vi "Check for Value Changes.vi"(8 "error in (no error)":errorcluster, 11 "Settings in":refnum<class "Settings.lvclass">) -> (0 "error out":errorcluster, 2 "Changes have been made":bool, 3 "Settings out":refnum<class "Settings.lvclass">)   [LabVIEW 2017, in "Settings.lvclass"]
uses:
  Settings.lvclass
  Settings.lvclass/Settings.ctl
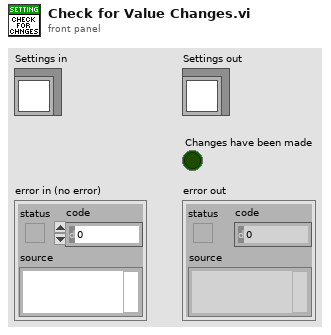
[diagram p1: front panel]
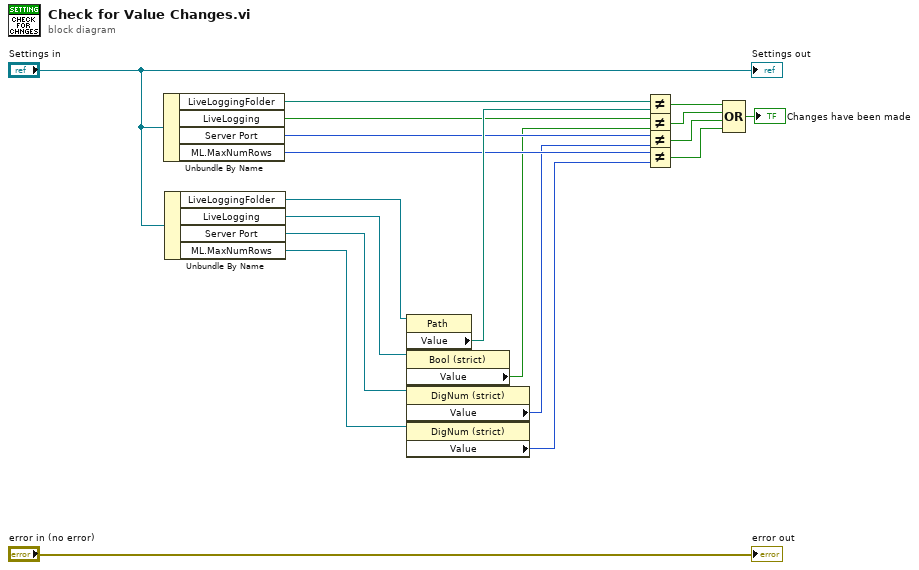
[diagram p0: block diagram]
diagram:
  n1 = Unbundle By Name("Settings in") -> ("LiveLoggingFolder"=w13:path, "LiveLogging"=w11:bool, "Server Port"=w10:u16, "ML.MaxNumRows"=w9:u16)
  n2 = Unbundle By Name("Settings in") -> ("LiveLoggingFolder"=w15:refnum<vi>, "LiveLogging"=w17:refnum<vi>, "Server Port"=w16:refnum<vi>, "ML.MaxNumRows"=w18:refnum<vi>)
  n3 = property class="Path"(reference=w15) -> ("Value"=w12:path)  [unwired: 1 in, 2 out]
  n4 = property class="Bool (strict)"(reference=w17) -> ("Value"=w8:bool)  [unwired: 1 in, 2 out]
  n5 = property class="DigNum (strict)"(reference=w16) -> ("Value"=w7:u16)  [unwired: 1 in, 2 out]
  n6 = property class="DigNum (strict)"(reference=w18) -> ("Value"=w6:u16)  [unwired: 1 in, 2 out]
  n7 = Not Equal?(x=w13, y=w12) -> (x != y?=w5:bool)
  n8 = Not Equal?(x=w11, y=w8) -> (x != y?=w4:bool)
  n9 = Not Equal?(x=w10, y=w7) -> (x != y?=w3:bool)
  n10 = Not Equal?(x=w9, y=w6) -> (x != y?=w2:bool)
  n11 = Compound Arithmetic op=OR(w5, w4, w3, w2) -> (→"Changes have been made":bool)
  "error out" <- "error in (no error)"
  "Settings out" <- "Settings in"
